vi "3.5.vi"() -> ()   [LabVIEW 2017]
panel:
  out "输出":dbl
  in  "输入":dbl
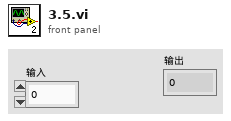
[diagram p1: front panel]
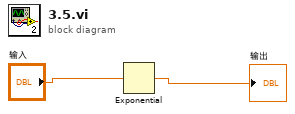
[diagram p0: block diagram]
diagram:
  n1 = Exponential(1:"输入") -> (0:→"输出":dbl)
